vi "nome_file.vi"(5 "numero file":i32, 7 "nome file":string, 10 "percorso iniziale":path=path "C:/Users/gioel/Koofr/università/tesi_magistrale/vi") -> (2 "risulato percorso":path)   [LabVIEW 2025]
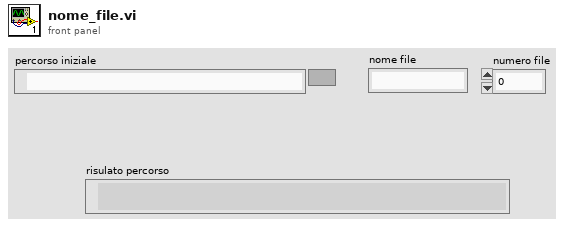
[diagram p1: front panel]
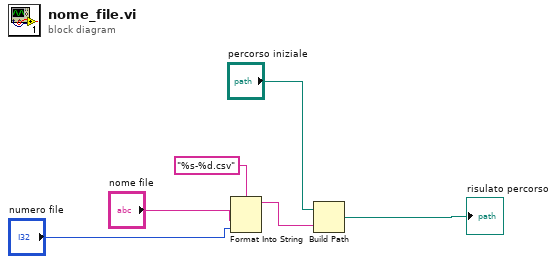
[diagram p0: block diagram]
diagram:
  n1 = Format Into String(format string="%s-%d.csv", "nome file", "numero file") -> (resulting string=w3:string)  [unwired: 2 in, 1 out]
  n2 = Build Path(base path="percorso iniziale", name or relative path=w3) -> (appended path=→"risulato percorso":path)
